vi "vna read meas.vi"(8 "error in (no error)":errorcluster, 9 "data format":T1, 10 "measurement name":string, 11 "VISA resource name":refnum<visa-resource-name>) -> (0 "error out":errorcluster, 2 "data":dbl[](array[numeric]), 3 "VISA resource name 2":refnum<visa-resource-name>)   [LabVIEW 2013]
uses:
  vna data formats.ctl
  vna block data type.ctl
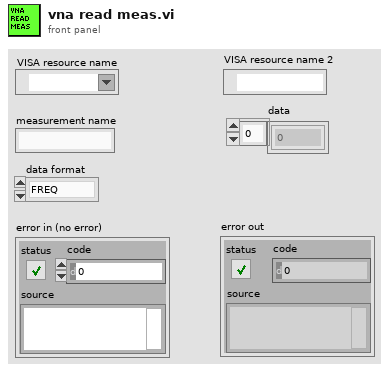
[diagram p1: front panel]
types:
  T1 = typedef "vna data formats.ctl" = enum16{"FREQ", "MLIN", "MLOG", "PHAS", "REAL", "IMAG"}
  T2 = typedef "vna block data type.ctl" = enum16{"REAL,32", "REAL,64"}
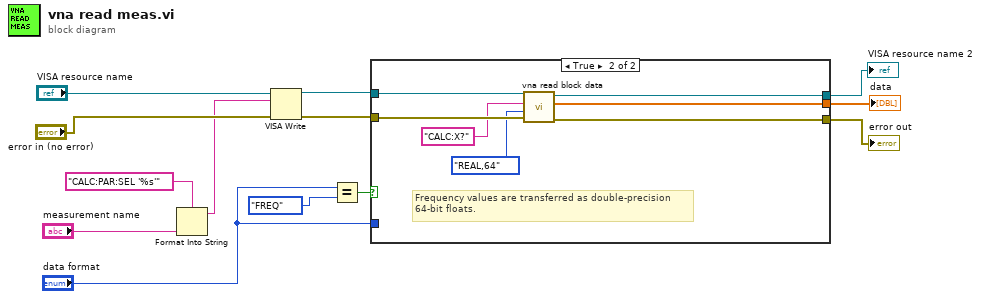
[diagram p0: block diagram]
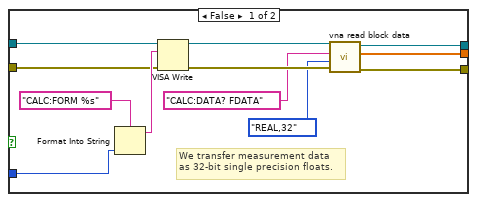
[diagram p2: hidden frame]
diagram:
  n1 = Format Into String(format string="CALC:PAR:SEL '%s'" ("write buffer"), "measurement name") -> (resulting string=w1:string)  [unwired: 2 in, 1 out]
  n2 = VISA Write(VISA resource name="VISA resource name", write buffer=w1, error in (no error)="error in (no error)") -> (VISA resource name out=w5:refnum<visa-resource-name>, error out=w4:errorcluster)  [unwired: 1 out]
  n3 = Equal?(x="data format", y=vna_data_formats."FREQ" ("data format")) -> (x = y?=w11:bool)
  n4 = case shown="True" w11 {
    tunnel: w5 -> [w23 w32]
    tunnel: w4 -> [w22 w31]
    tunnel: [w17 w28] -> w7
    tunnel: [w16 w27] -> w9
    tunnel: [w15 w26] -> w8
    tunnel: "data format" -> [w14 _]
    frame False {
      # "We transfer measurement data \nas 32-bit single precision floats."
      n5 = Format Into String(format string="CALC:FORM %s" ("write buffer"), w14) -> (resulting string=w24:string)  [unwired: 2 in, 1 out]
      n6 = VISA Write(VISA resource name=w23, write buffer=w24, error in (no error)=w22) -> (VISA resource name out=w20:refnum<visa-resource-name>, error out=w21:errorcluster)  [unwired: 1 out]
      n7 = call "vna read block data.vi"("error in (no error)"=w21, "data type"=vna_block_data_type."REAL,32", "command"="CALC:DATA? FDATA", "VISA resource name"=w20) -> ("error out"=w17:errorcluster, "data"=w15:dbl[], "VISA resource name"=w16:refnum<visa-resource-name>)  [unwired: 5 in]
    }
    frame True {
      # "Frequency values are transferred as double-precision\n64-bit floats."
      n8 = call "vna read block data.vi"("error in (no error)"=w31, "data type"=vna_block_data_type."REAL,64", "command"="CALC:X?", "VISA resource name"=w32) -> ("error out"=w28:errorcluster, "data"=w26:dbl[], "VISA resource name"=w27:refnum<visa-resource-name>)  [unwired: 5 in]
    }
  }
  "VISA resource name 2" <- w9
  "error out" <- w7
  "data" <- w8
